vi "Error_Log_Close.vi"(8 "error in (no error)":errorcluster) -> (0 "error out":errorcluster)   [LabVIEW 2011]
uses:
  <userlib>/_JGCODE/error_logger/_error_logger.llb/ErrorLogger.lvclass
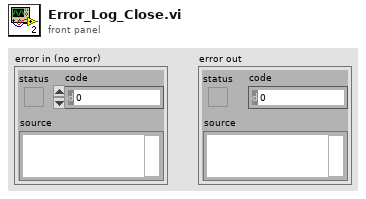
[diagram p1: front panel]
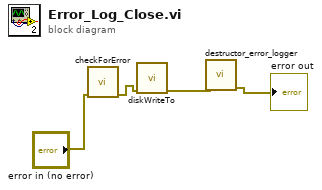
[diagram p0: block diagram]
diagram:
  n1 = call <userlib>:"checkForError.vi"("Error In"="error in (no error)") -> ("error out"=w1:errorcluster)  [unwired: 9 in, 1 out]
  n2 = call <userlib>:"diskWriteTo.vi"("error in (no error)"=w1) -> ("error out"=w2:errorcluster)  [unwired: 10 in]
  n3 = call <userlib>:"destructor_error_logger.vi"("error in (no error)"=w2) -> ("error out"=→"error out":errorcluster)  [unwired: 10 in]
